vi "B-Scan (LLC messages) DVR.vi"(7 "Micropulse # In":i32, 9 "Scan definition":T1={"Scan Start"=0.0, "Scan Length"=280.0, "Inspection Resolution"=0.5, "Direction"=enum."Forwards"} {"Inspection Resolution" format="%#_6f"; "Scan Start" format="%#_6f"; "Scan Length" format="%#_6f"}, 10 "Axis No.":u8=1 min=1 max=4, 11 "scan data info":T3 {"Error Message" format="%04x"; "Message Header" format="%04x"; "IP"."MIP location" format="%#.0f"; "IP"."Location" format="%#.0f"; "PRF" format="%.0fHz"}) -> (0 "Update Display?":bool, 1 "B-Scan In Progress?":bool, 2 "B-Scan index":i32, 3 "data value reference":refnum<data-value>)   [LabVIEW 2026, in "MicroPulse_Driver.lvlib"]
uses:
  MicroPulse_Driver.lvlib
  Data/Datatypes/MP - scan data info.ctl
  Data/Datatypes/MP - data output format.ctl
  Data/Datatypes/MP - retain scan.ctl
  Data/Datatypes/MP - axis positions (LLC).ctl
  Data/Datatypes/MP - fly scan range.ctl
  Data/Datatypes/MP - inspection direction.ctl
  Low Level/FGV - B-Scan Active - Action [Enum].ctl
  <instrlib>/Micropulse/Micropulse.lvlib
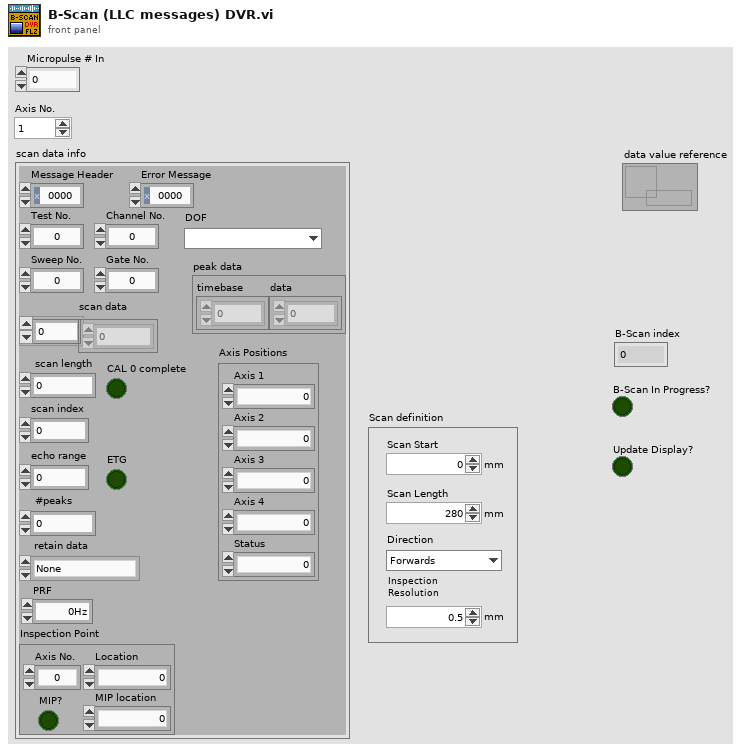
[diagram p1: front panel]
types:
  T1 = typedef "Micropulse.lvlib/MP - fly scan range.ctl" = cluster{"Scan Start":dbl, "Scan Length":dbl, "Inspection Resolution":dbl, "Direction":T2}
  T2 = typedef "Micropulse.lvlib/MP - inspection direction.ctl" = enum16{"Forwards", "Backwards"}
  T3 = typedef "Micropulse.lvlib/MP - scan data info.ctl" = cluster{"Message Header":u16, "Error Message":u16, "Test No.":u32, "Channel No.":u8, "Sweep No.":u32, "Gate No.":u32, "DOF":T4, "retain data":T5, "scan data":u16[], "scan length":i32, "scan index":i32, "peak data":cluster{"timebase":u16[], "data":u16[]}, "#peaks":i32, "PRF":dbl, "IP":cluster{"Axis No.":u8, "Location":u32, "MIP location":u32, "MIP?":bool}, "echo range":u16, "ETG":bool, "CAL 0 complete":bool, "Axis Positions":T6}
  T4 = typedef "Micropulse.lvlib/MP - data output format.ctl" = enum16{"", "8-bit Mode", "10-bit Mode", "12-bit Mode", "16-bit Mode", "8-bit Log Mode", "12-bit Packed Mode"}
  T5 = typedef "Micropulse.lvlib/MP - retain scan.ctl" = enum16{"None", "Ascan", "Peaks"}
  T6 = typedef "Micropulse.lvlib/MP - axis positions (LLC).ctl" = cluster{"Axis 1":u32, "Axis 2":u32, "Axis 3":u32, "Axis 4":u32, "Status":u8}
  T7 = typedef "MicroPulse_Driver.lvlib/FGV - B-Scan Active - Action [Enum].ctl" = enum16{"Read", "Read & Reset Start Flag", "Start B-Scan", "B-Scan Finished"}
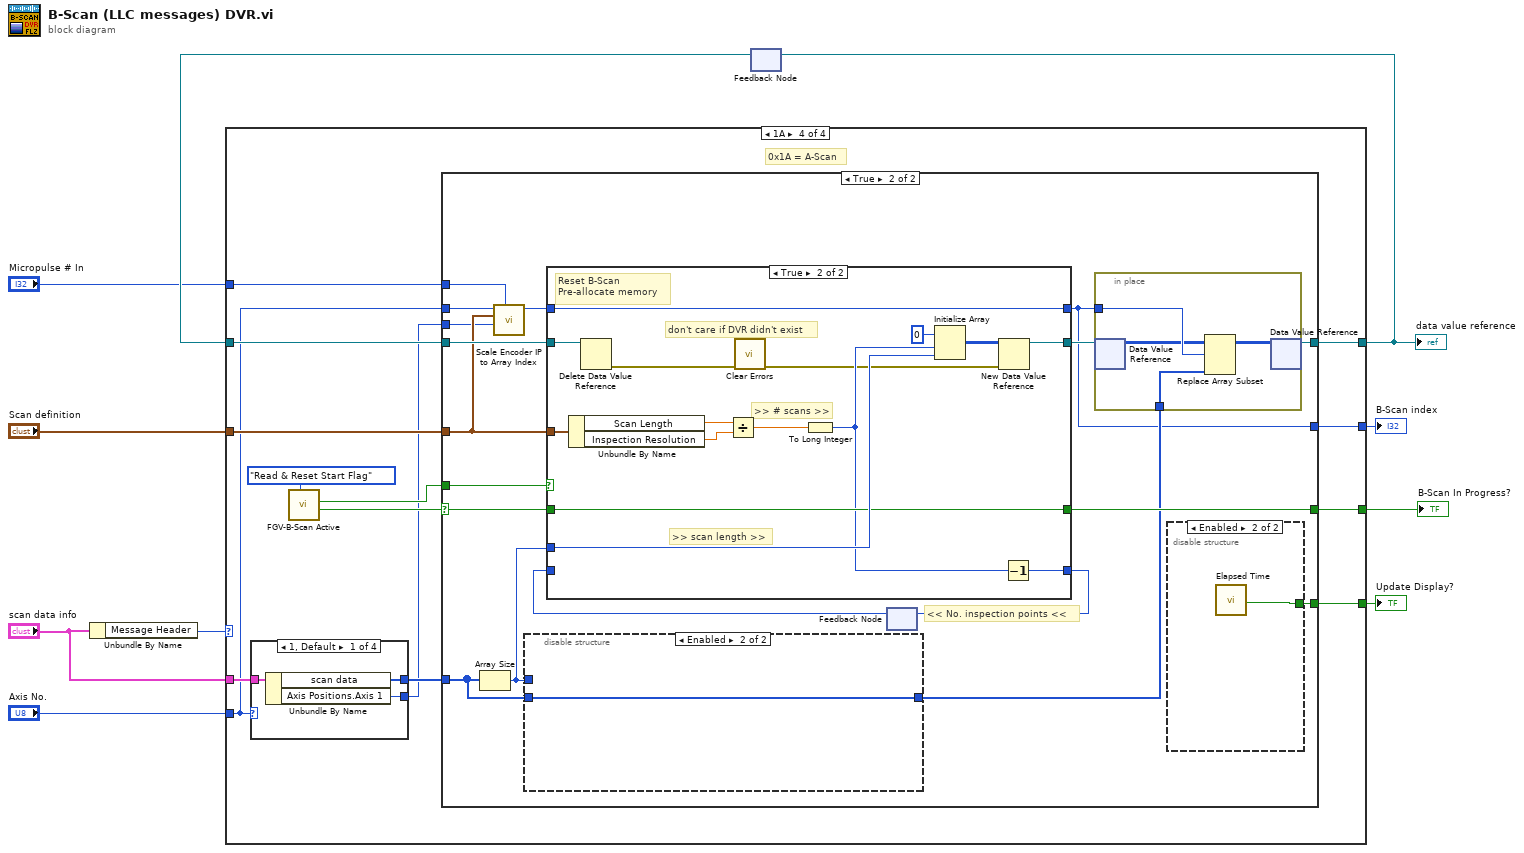
[diagram p0: block diagram]
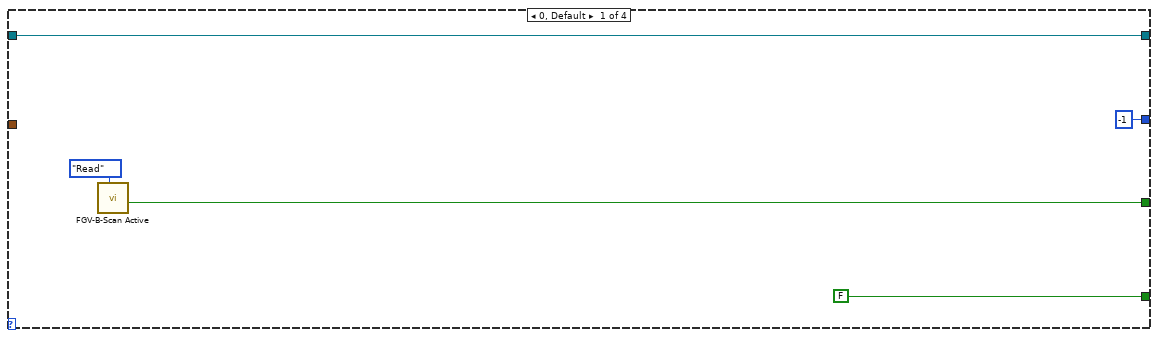
[diagram p2: hidden frame]
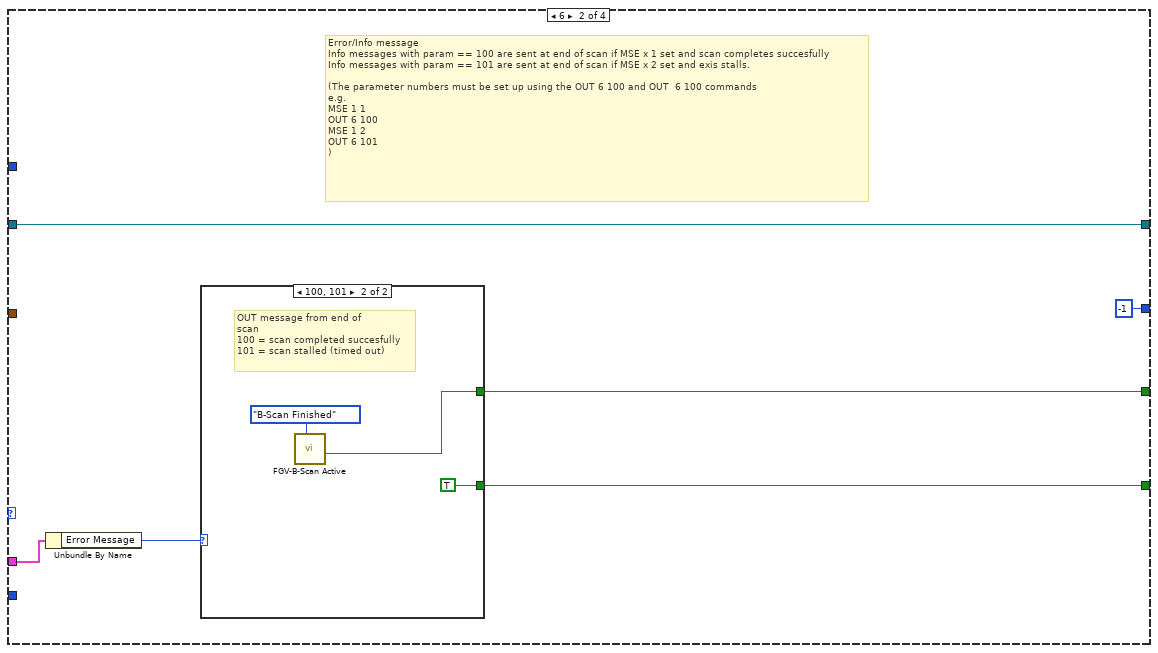
[diagram p3: hidden frame]
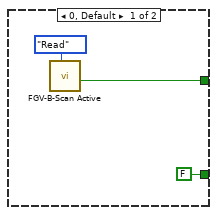
[diagram p4: hidden frame]
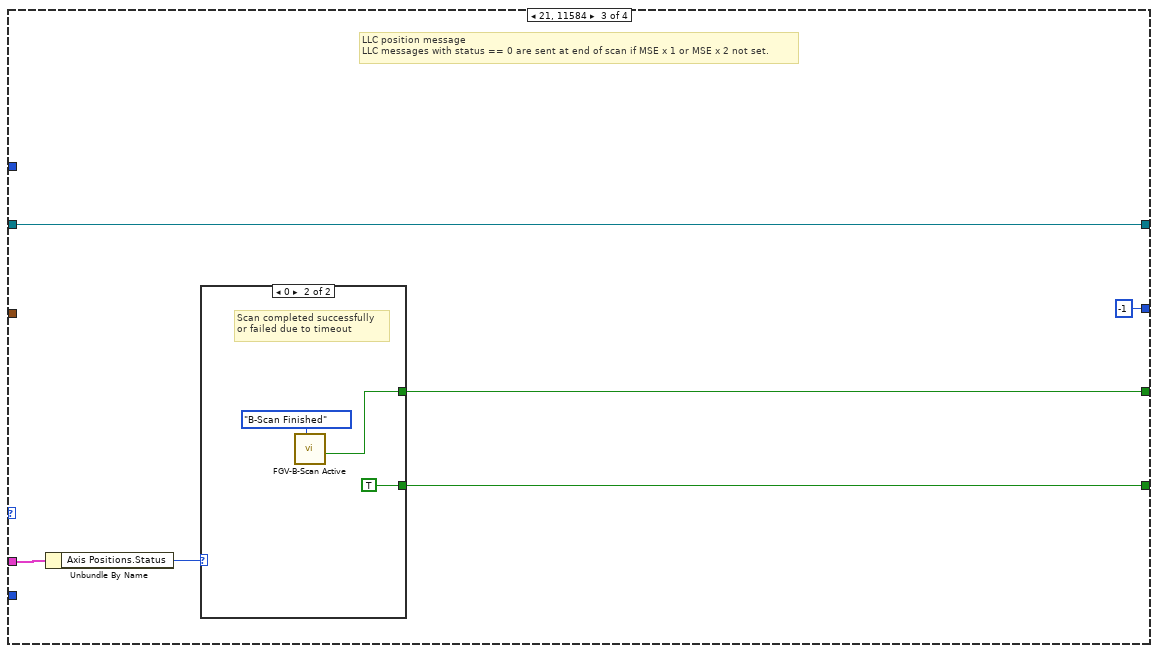
[diagram p5: hidden frame]
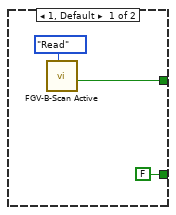
[diagram p6: hidden frame]
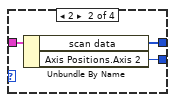
[diagram p7: hidden frame]
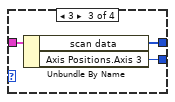
[diagram p8: hidden frame]
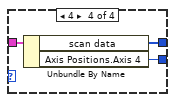
[diagram p9: hidden frame]
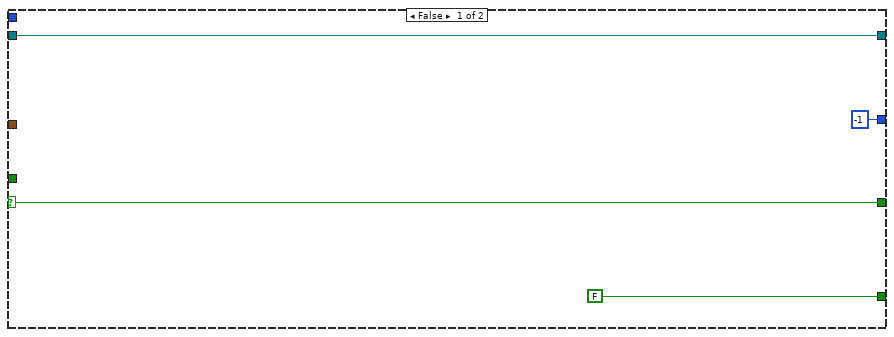
[diagram p10: hidden frame]
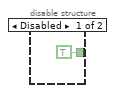
[diagram p11: hidden frame]
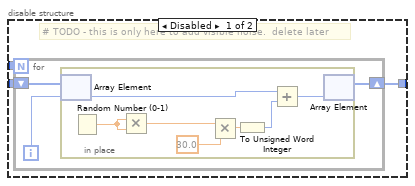
[diagram p12: hidden frame]
diagram:
  n1 = Unbundle By Name("scan data info") -> ("Message Header"=w10:u16)
  n2 = feedback #1() -> (w6:refnum<data-value>)  [unwired: 1 in]
  n3 = case shown="1A" w10 {
    tunnel: "scan data info" -> [_ w20 w32 w53]
    tunnel: "Scan definition" -> [_ _ _ w47]
    tunnel: [w15 w21 w33 w51] -> w7
    tunnel: w6 -> [w15 w21 w33 w50]
    tunnel: "Micropulse # In" -> [_ _ _ w46]
    tunnel: [w12 w18 w30 w49] -> w4
    tunnel: [FALSE w16 w28 w48] -> w3
    tunnel: "Axis No." -> [_ _ _ w41]
    tunnel: [-1 ("B-Scan index") -1 ("B-Scan index") -1 ("B-Scan index") w40] -> w1
    frame 0, Default {
      n4 = call "FGV-B-Scan Active.vi"("Action"=FGV_-_B-Scan_Active_-_Action_[Enum]."Read") -> ("B-Scan In Progress?"=w12:bool)  [unwired: 8 in, 2 out]
    }
    frame 6 {
      # "Error/Info message\nInfo messages with param == 100 are sent at end of scan if MSE x 1 set and scan completes succesfully\nInfo messages with param == 101 are sent at end of scan if MSE x 2 set and exis stalls.\n\n(The parameter numbers must be set up using the OUT 6 100 and OUT  6 100 commands \ne.g.\nMSE 1 1\nOUT 6 100\nMSE 1 2\nOUT 6 101\n)"
      n5 = Unbundle By Name(w20) -> ("Error Message"=w19:u16)
      n6 = case shown="100, 101" w19 {
        tunnel: [w23 w26] -> w18
        tunnel: [FALSE TRUE] -> w16
        frame 0, Default {
          n7 = call "FGV-B-Scan Active.vi"("Action"=FGV_-_B-Scan_Active_-_Action_[Enum]."Read") -> ("B-Scan In Progress?"=w23:bool)  [unwired: 8 in, 2 out]
        }
        frame 100, 101 {
          # "OUT message from end of\nscan\n100 = scan completed succesfully\n101 = scan stalled (timed out)"
          n8 = call "FGV-B-Scan Active.vi"("Action"=FGV_-_B-Scan_Active_-_Action_[Enum]."B-Scan Finished") -> ("B-Scan In Progress?"=w26:bool)  [unwired: 8 in, 2 out]
        }
      }
    }
    frame 21, 11584 {
      # "LLC position message\nLLC messages with status == 0 are sent at end of scan if MSE x 1 or MSE x 2 not set."
      n9 = Unbundle By Name(w32) -> ("Axis Positions.Status"=w31:u8)
      n10 = case shown="0" w31 {
        tunnel: [w35 w38] -> w30
        tunnel: [FALSE TRUE] -> w28
        frame 1, Default {
          n11 = call "FGV-B-Scan Active.vi"("Action"=FGV_-_B-Scan_Active_-_Action_[Enum]."Read") -> ("B-Scan In Progress?"=w35:bool)  [unwired: 8 in, 2 out]
        }
        frame 0 {
          # "Scan completed successfully\nor failed due to timeout"
          n12 = call "FGV-B-Scan Active.vi"("Action"=FGV_-_B-Scan_Active_-_Action_[Enum]."B-Scan Finished") -> ("B-Scan In Progress?"=w38:bool)  [unwired: 8 in, 2 out]
        }
      }
    }
    frame 26 {
      # "0x1A = A-Scan"
      n13 = case shown="1, Default" w41 {
        tunnel: w53 -> [w56 w59 w62 w65]
        tunnel: [w55 w58 w61 w64] -> w52
        tunnel: [w54 w57 w60 w63] -> w42
        frame 1, Default {
          n14 = Unbundle By Name(w56) -> ("scan data"=w55:u16[], "Axis Positions.Axis 1"=w54:u32)
        }
        frame 2 {
          n15 = Unbundle By Name(w59) -> ("scan data"=w58:u16[], "Axis Positions.Axis 2"=w57:u32)
        }
        frame 3 {
          n16 = Unbundle By Name(w62) -> ("scan data"=w61:u16[], "Axis Positions.Axis 3"=w60:u32)
        }
        frame 4 {
          n17 = Unbundle By Name(w65) -> ("scan data"=w64:u16[], "Axis Positions.Axis 4"=w63:u32)
        }
      }
      n18 = call "FGV-B-Scan Active.vi"("Action"=FGV_-_B-Scan_Active_-_Action_[Enum]."Read & Reset Start Flag") -> ("B-Scan In Progress?"=w43:bool, "B-Scan Start?"=w44:bool)  [unwired: 8 in, 1 out]
      n19 = case shown="True" w43 {
        selector: w43 -> [w68 w83]
        tunnel: w50 -> [w69 w87]
        tunnel: [w69 w71] -> w51
        tunnel: w52 -> [_ w78]
        tunnel: w47 -> [_ w75]
        tunnel: [w68 w84] -> w49
        tunnel: [FALSE w82] -> w48
        tunnel: w46 -> [_ w79]
        tunnel: w44 -> [_ w76]
        tunnel: w42 -> [_ w74]
        tunnel: w41 -> [_ w73]
        tunnel: [-1 ("B-Scan index") w70] -> w40
        frame False {
        }
        frame True {
          # "<< No. inspection points <<"
          n20 = Array Size(array=w78) -> (size(s)=w77:i32)
          n21 = call "Scale Encoder IP to Array Index.vi"("Micropulse # In"=w79, "Inspection Point Location"=w74, "Scan definition"=w75, "Axis No."=w73) -> ("B-Scan index"=w80:i32)  [unwired: 6 in, 1 out]
          n22 = disable-structure shown="Enabled" {
            disable-tunnel: [w96 w107] -> w81
            disable-tunnel: w78 -> [w95 w107]
            disable-tunnel: w77 -> [w94 _]
            frame Disabled {
              # "# TODO - this is only here to add visible noise.  delete later"
              n23 = for {
                N: w94 -> [_]
                shift-right: [w97] -> w96
                shift-left: w95 -> [w99]
                i -> [w98]
                n24 = in-place {
                  n25 = in-place-array #2(w99, w98) -> (w103:u16)
                  n26 = Random Number (0-1)() -> (number: 0 to 1=w100:dbl)
                  n27 = Multiply(x=w100, y=w100) -> (x*y=w101:dbl)
                  n28 = Multiply(x=w101, y=30.0) -> (x*y=w105:dbl)
                  n29 = To Unsigned Word Integer(number=w105) -> (unsigned 16bit integer=w104:u16)
                  n30 = Add(x=w103, y=w104) -> (x+y=w102:u16)
                  n31 = in-place-array #2(w102) -> (w97:u16[])  [unwired: 1 out]
                }
              }
            }
            frame Enabled {
            }
          }
          n32 = feedback #3() -> (w85:i32)  [unwired: 1 in]
          n33 = case shown="True" w76 {
            tunnel: w87 -> [w111 w114]
            tunnel: [w111 w115] -> w72
            tunnel: w75 -> [_ w125]
            tunnel: w77 -> [_ w122]
            tunnel: w80 -> [w109 w118]
            tunnel: [w108 w121] -> w86
            tunnel: w85 -> [w108 _]
            tunnel: [w110 w119] -> w84
            tunnel: w83 -> [w110 w119]
            tunnel: [w109 w118] -> w70
            frame False {
            }
            frame True {
              # "don't care if DVR didn't exist"
              # "Reset B-Scan\nPre-allocate memory"
              # ">> scan length >>"
              # ">> # scans >>"
              n34 = Unbundle By Name(w125) -> ("Scan Length"=w124:dbl, "Inspection Resolution"=w123:dbl)
              n35 = Delete Data Value Reference(data value reference=w114) -> (error out=w113:errorcluster)  [unwired: 1 in, 1 out]
              n36 = Divide(x=w124, y=w123) -> (x/y=w120:dbl)
              n37 = call <vilib>:"Clear Errors.vi"("error in (no error)"=w113) -> ("error out"=w112:errorcluster)  [unwired: 5 in, 1 out]
              n38 = To Long Integer(number=w120) -> (32bit integer=w117:i32)
              n39 = Initialize Array(u16 0 ("index"), w117, w122) -> (w116:u16[][])
              n40 = New Data Value Reference(data value=w116, error in=w112) -> (data value reference=w115:refnum<data-value>)  [unwired: 1 out]
              n41 = Decrement(x=w117) -> (x-1=w121:i32)
            }
          }
          n42 = feedback-in #3(w86) -> ()
          n43 = in-place {
            in-place-border: w81 -> [w91]
            in-place-border: w70 -> [w90]
            n44 = in-place-dvr #4(w72) -> (w89:u16[][])  [unwired: 1 out]
            n45 = Replace Array Subset(array=w89, new element=w91, index (row)=w90) -> (w88:u16[][])  [unwired: 1 in]
            n46 = in-place-dvr #4(w88) -> (w71:refnum<data-value>)  [unwired: 1 out]
          }
          n47 = disable-structure shown="Enabled" {
            disable-tunnel: [TRUE w93] -> w82
            frame Disabled {
            }
            frame Enabled {
              n48 = call "Elapsed Time"() -> ("Time has Elapsed"=w93:bool)  [unwired: 12 in, 7 out]
            }
          }
        }
      }
    }
  }
  "Update Display?" <- w3
  "B-Scan In Progress?" <- w4
  "B-Scan index" <- w1
  "data value reference" <- w7
  n49 = feedback-in #1(w7) -> ()
